vi "Analyze IQ.vi"(8 "error in (no error)":errorcluster, 11 "wfm dat":waveform(cdb)) -> (0 "error out":errorcluster, 1 "Seconds to Analyze":dbl, 2 "Bytes Analyzed":i32 format="%.1pB", 3 "Power Spectrum":cluster{"f0":dbl, "df":dbl, "magnitude":dbl[]} {"magnitude" format="%.2p"; "f0" format="%0.2p"; "df" format="%0.2p"}, 5 "Bytes Analyzed per Second":dbl format="%#_5pB/sec")   [LabVIEW 2021]
uses:
  <vilib>/measure/maspectr.llb/FFT Power Spectrum and PSD for 1 Chan (CDB).vi
  <vilib>/measure/NI_MAPro.lvlib
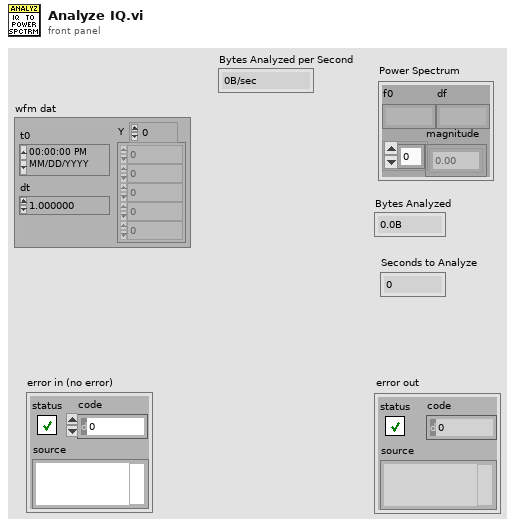
[diagram p1: front panel]
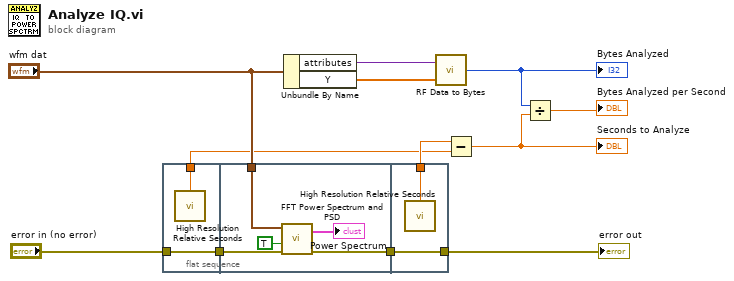
[diagram p0: block diagram]
diagram:
  n1 = flat-sequence {
    tunnel: [w14] -> w7
    tunnel: "error in (no error)" -> [w14]
    tunnel: [w13] -> w2
    tunnel: "wfm dat" -> [w17]
    tunnel: w7 -> [w16]
    tunnel: [w15] -> w6
    tunnel: w6 -> [w21]
    tunnel: [w21] -> w9
    tunnel: [w20] -> w3
    frame #0 {
      n2 = call <vilib>:"High Resolution Relative Seconds.vi"() -> ("relative seconds"=w13:dbl)
    }
    frame #1 {
      n3 = call-poly <vilib>:"FFT Power Spectrum and PSD.vi"("error in (no error)"=w16, "dB On (F)"=TRUE, "time signal"=w17) -> ("error out"=w15:errorcluster, "Power Spectrum / PSD"=→"Power Spectrum":cluster{"f0":dbl, "df":dbl, "magnitude":dbl[]})  [unwired: 5 in, 2 out]
    }
    frame #2 {
      n4 = call <vilib>:"High Resolution Relative Seconds.vi"() -> ("relative seconds"=w20:dbl)
    }
  }
  n5 = Unbundle By Name("wfm dat") -> ("attributes"=w5:variant, "Y"=w4:cdb[])
  n6 = call "RF Data to Bytes.vi"("Y"=w4, "attributes"=w5) -> ("Bytes"=w11:i32)
  "Bytes Analyzed" <- w11
  n7 = Subtract(x=w3, y=w2) -> (x-y=w1:dbl)
  "Seconds to Analyze" <- w1
  n8 = Divide(x=w11, y=w1) -> (x/y=→"Bytes Analyzed per Second":dbl)
  "error out" <- w9
